vi "UTILITY Semaphore Create Local.vi"(3 "Semiphore":T1, 5 "error in (no error)":errorcluster, 9 "name (unnamed)":string) -> (17 "semaphore":T1, 18 "Local?":bool, 19 "error out":errorcluster)   [LabVIEW 2016]
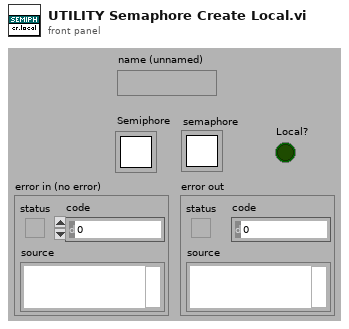
[diagram p1: front panel]
types:
  T1 = typedef "Semaphore RefNum" = refnum<k1>
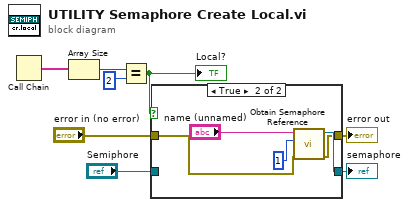
[diagram p0: block diagram]
diagram:
  n1 = Call Chain() -> (call chain=w6:string[])
  n2 = Array Size(array=w6) -> (size(s)=w7:i32)
  n3 = Equal?(x=w7, y=2) -> (x = y?=w5:bool)
  "Local?" <- w5
  n4 = case shown="True" w5 {
    tunnel: [w9 w14] -> w1
    tunnel: "error in (no error)" -> [w10 w13]
    tunnel: [w10 w12] -> w2
    tunnel: "Semiphore" -> [w9 _]
    frame False {
    }
    frame True {
      n5 = call <vilib>:"Obtain Semaphore Reference.vi"("error in (no error)"=w13, "size (1)"=1, "name (unnamed)"="name (unnamed)") -> ("error out"=w12:errorcluster, "semaphore"=w14:T1)  [unwired: 2 in, 1 out]
    }
  }
  "error out" <- w2
  "semaphore" <- w1
